vi "Fetch VI Method Info.vi"(7 "Fetch FP Info? (F)":bool, 8 "Error in":errorcluster caption="Error in (no error)", 9 "Dispatch (None)":T4, 10 "VI Reference":refnum<vi>, 11 "VI ProjectItem in":refnum<vi>) -> (0 "Error out":errorcluster, 3 "Method Spec Cluster":T1)   [LabVIEW 2023, in "VIDoc Parsing.lvlib"]
uses:
  VIDoc Parsing.lvlib
  TypeDefs/Class Dispatch Type Enum.ctl
  TypeDefs/Method Spec Cluster.ctl
  TypeDefs/VI Type Extended Enum.ctl
  <vilib>/picture/picture.llb/imagedata.ctl
  TypeDefs/Controls Info Cluster.ctl
  <vilib>/Utility/miscctls.llb/LVKeyTypeDef.ctl
  <vilib>/Utility/miscctls.llb/LVPointTypeDef.ctl
  Structure Reporter/Tree Cluster.ctl
  Structure Reporter/Structure Reporter.lvlib
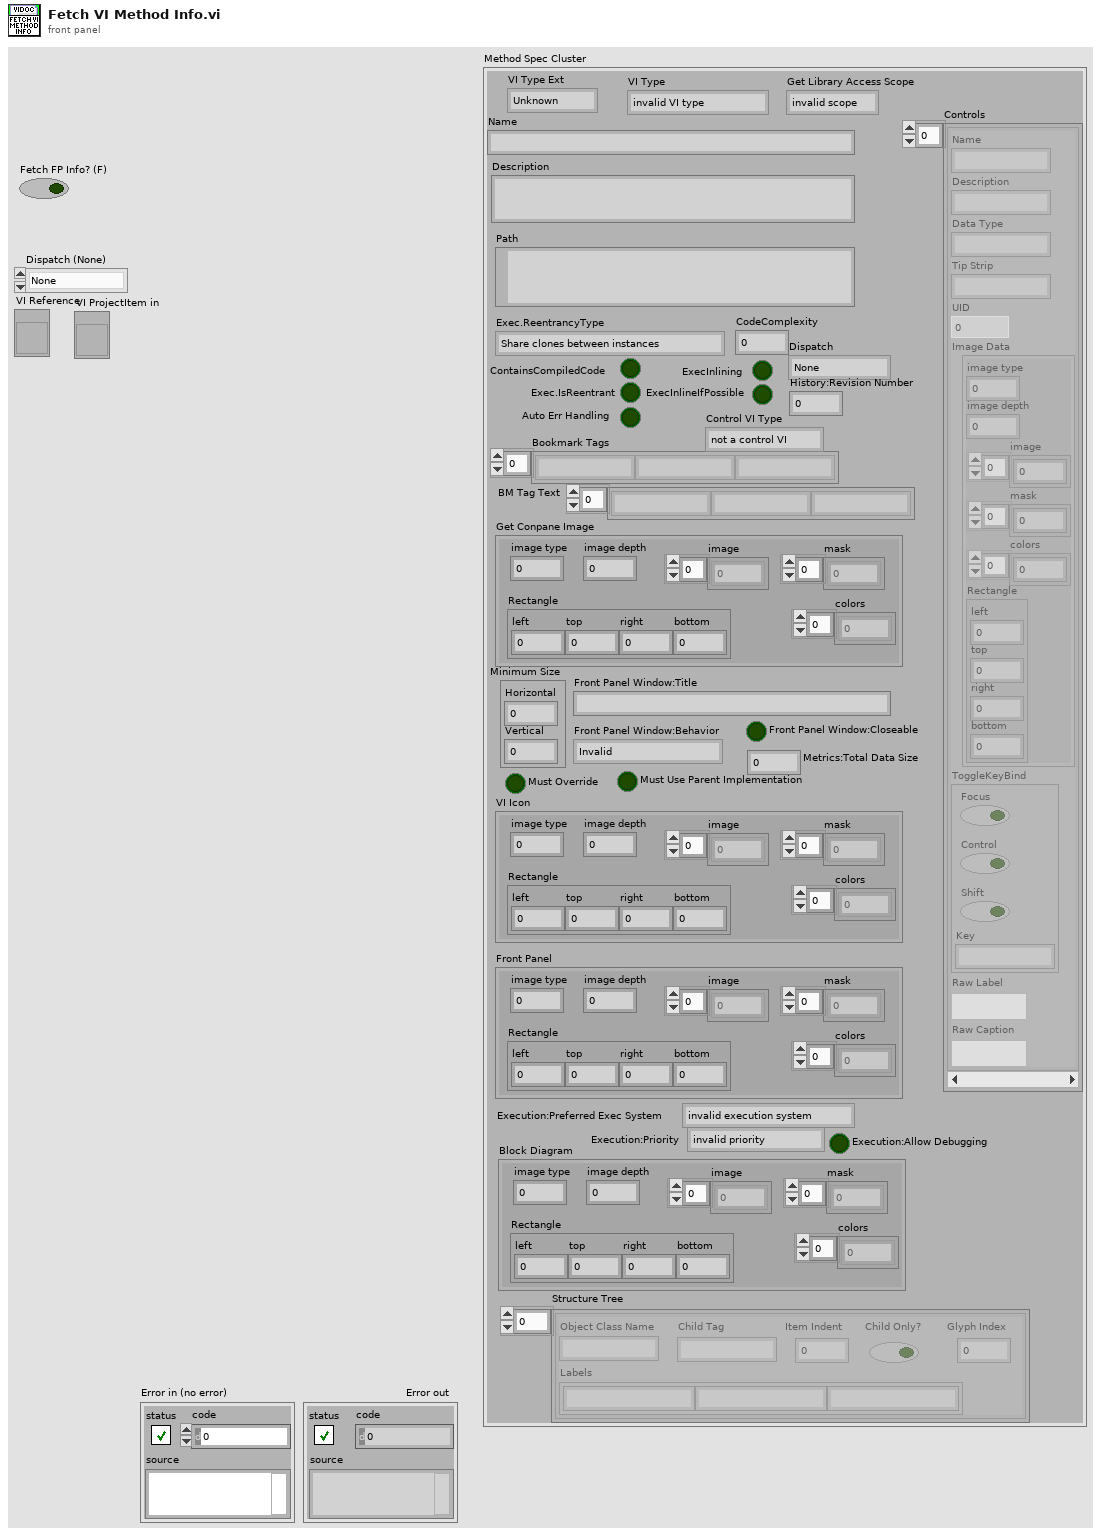
[diagram p1: front panel]
types:
  T1 = typedef "VIDoc Parsing.lvlib/Method Spec Cluster.ctl" = cluster{"VI Type Ext":T2, "Name":string, "Path":path, "Get Conpane Image":T3, "Description":string, "Get Library Access Scope":enum32{"invalid scope", "public", "private", "protected", "community"}, "Dispatch":T4, "ContainsCompiledCode":bool, "Exec.IsReentrant":bool, "Exec.ReentrancyType":enum16{"Share clones between instances", "Preallocate clone for each instance"}, "ExecInlining":bool, "ExecInlineIfPossible":bool, "Auto Err Handling":bool, "CodeComplexity":sgl, "Bookmark Tags":string[], "Control VI Type":enum32{"not a control VI", "control", "typedef", "strict typedef"}, "Controls":T5[], "VI Type":enum32{"invalid VI type", "Standard VI", "Control VI", "Global VI", "Polymorphic VI", "Configuration VI", "SubSystem", "Facade VI", "Method VI", "Statechart Diagram VI"}, "Minimum Size":T7, "Front Panel Window:Title":string, "Front Panel Window:Behavior":enum32{"Invalid", "Default", "Floating", "Floating/Auto-Hide", "Modal"}, "Front Panel Window:Closeable":bool, "Must Override":bool, "Must Use Parent Implementation":bool, "VI Icon":T3, "Front Panel":T3, "History:Revision Number":u32, "Metrics:Total Data Size":u32, "Execution:Allow Debugging":bool, "Execution:Preferred Exec System":enum32{"invalid execution system", "user interface", "standard", "instrument i/o", "data acquisition", "other 1", "other 2", "same as caller"}, "Execution:Priority":enum32{"invalid priority", "background priority", "normal priority", "above normal priority", "high priority", "time critical priority", "subroutine"}, "BM Tag Text":string[], "Block Diagram":T3, "Structure Tree":T8[]}
  T2 = typedef "VIDoc Parsing.lvlib/VI Type Extended Enum.ctl" = enum16{"Unknown", "Class Method", "Class Accessor Get", "Class Accessor Set", "Class Control", "Library Method", "Library Control", "VI", "Control"}
  T3 = typedef "imagedata.ctl" = cluster{"image type":i32, "image depth":i32, "image":u8[], "mask":u8[], "colors":u32[], "Rectangle":cluster{"left":i16, "top":i16, "right":i16, "bottom":i16}}
  T4 = typedef "VIDoc Parsing.lvlib/Class Dispatch Type Enum.ctl" = enum16{"None", "Static", "Dynamic"}
  T5 = typedef "VIDoc Parsing.lvlib/Controls Info Cluster.ctl" = cluster{"Name":string, "Description":string, "Data Type":string, "Tip Strip":string, "UID":i32, "Image Data":T3, "ToggleKeyBind":T6, "Raw Label":string, "Raw Caption":string}
  T6 = typedef "LVKeyTypeDef.ctl" = cluster{"Focus":bool, "Control":bool, "Shift":bool, "Key":string}
  T7 = typedef "LVPointTypeDef.ctl" = cluster{"Horizontal":i16, "Vertical":i16}
  T8 = typedef "VIDoc Parsing.lvlib/Structure Reporter.lvlib/Tree Cluster.ctl" = cluster{"Object Class Name":string, "Labels":string[], "Child Tag":string, "Item Indent":i32, "Child Only?":bool, "Glyph Index":i32}
  T9 = enum32{"not a control VI", "control", "typedef", "strict typedef"}
  T10 = enum16{"Share clones between instances", "Preallocate clone for each instance"}
  T11 = enum32{"invalid execution system", "user interface", "standard", "instrument i/o", "data acquisition", "other 1", "other 2", "same as caller"}
  T12 = enum32{"invalid priority", "background priority", "normal priority", "above normal priority", "high priority", "time critical priority", "subroutine"}
  T13 = enum32{"invalid scope", "public", "private", "protected", "community"}
  T14 = typedef "LVBookmarkInfoTypeDef.ctl" = cluster{"Bookmark ID":u32, "Bookmark Tag":string, "Label Text":string}[]
  T15 = typedef "VIDoc Parsing.lvlib/Structure Reporter.lvlib/Structure Result 2.ctl" = cluster{"Depth":i32, "Top":i32, "Left":i32, "Frame index":i32, "Struct":i32, "Object Class Name":string, "Object UID":i32, "Label Visible":bool, "Object Label":string, "SD Label Visible":bool, "Object SD Label":string, "Frame Name":string, "Diag UID":i32, "Owner Class Name":string, "Owner UID":i32, "Diag Struct":i32[], "Parent Struct":i32, "Diag UIDs":i32[], "Tree Name":string, "Diag Ref":refnum<vi>, "Owner Classes":string[], "Owner":refnum<vi>, "Owner UIDs":i32[], "Tag Indent":i32, "Tag Value":i32, "Child Tag":string}
  T16 = enum32{"Invalid", "Default", "Floating", "Floating/Auto-Hide", "Modal"}
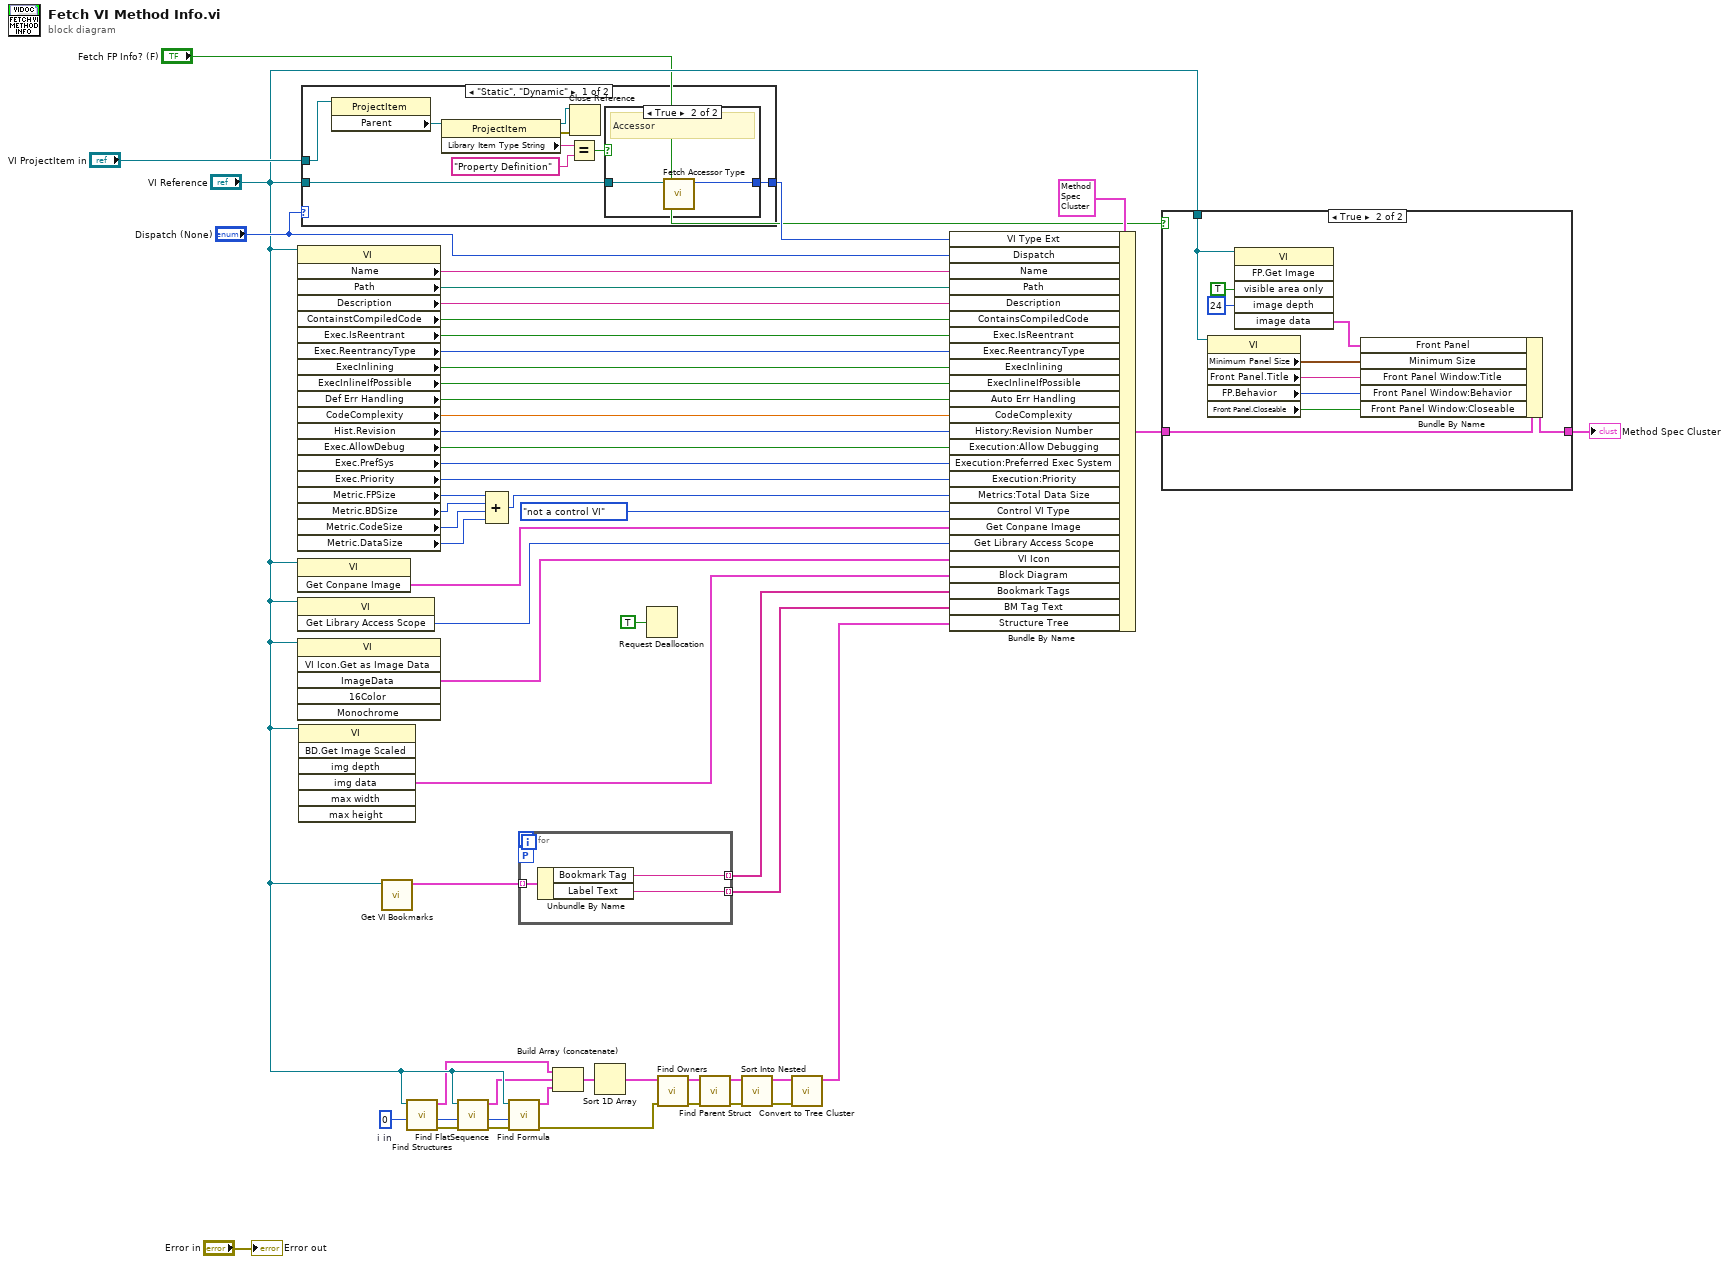
[diagram p0: block diagram]
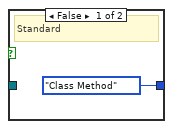
[diagram p3: hidden frame]
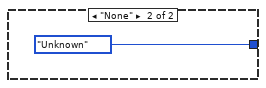
[diagram p4: hidden frame]
diagram:
  w17 = 0  # i in
  n1 = property class="VI"(reference="VI Reference") -> ("Name"=w48:string, "Path"=w47:path, "Description"=w46:string, "ContainstCompiledCode"=w45:bool, "Exec.IsReentrant"=w44:bool, "Exec.ReentrancyType"=w43:T10, "ExecInlining"=w42:bool, "ExecInlineIfPossible"=w41:bool, "Def Err Handling"=w40:bool, "CodeComplexity"=w39:sgl, "Hist.Revision"=w38:u32, "Exec.AllowDebug"=w37:bool, "Exec.PrefSys"=w36:T11, "Exec.Priority"=w35:T12, "Metric.FPSize"=w53:u32, "Metric.BDSize"=w52:u32, "Metric.CodeSize"=w51:u32, "Metric.DataSize"=w50:u32)  [unwired: 1 in, 2 out]
  n2 = invoke class="VI" method="Get Conpane Image"(reference="VI Reference") -> ("Get Conpane Image"=w33:T3)  [unwired: 2 in, 2 out]
  n3 = invoke class="VI" method="Get Library Access Scope"(reference="VI Reference") -> ("Get Library Access Scope"=w32:T13)  [unwired: 2 in, 2 out]
  n4 = invoke class="VI" method="VI Icon.Get as Image Data"(reference="VI Reference") -> ("ImageData"=w31:T3)  [unwired: 5 in, 5 out]
  n5 = invoke class="VI" method="BD.Get Image Scaled"(reference="VI Reference") -> ("img data"=w21:T3)  [unwired: 6 in, 6 out]
  n6 = case shown="\"Static\", \"Dynamic\"" "Dispatch (None)" {
    tunnel: "VI ProjectItem in" -> [w64 _]
    tunnel: [w60 VI_Type_Extended_Enum."Unknown" ("VI Type Ext")] -> w28
    tunnel: "VI Reference" -> [w58 _]
    frame "Static", "Dynamic" {
      n7 = property class="ProjectItem"(reference=w64) -> ("Parent"=w61:refnum<vi>)  [unwired: 1 in, 2 out]
      n8 = property class="ProjectItem"(reference=w61) -> (reference out=w56:refnum<vi>, error out=w57:errorcluster, "Library Item Type String"=w62:string)  [unwired: 1 in]
      n9 = Equal?(x=w62, y="Property Definition") -> (x = y?=w59:bool)
      n10 = Close Reference(reference=w56, error in (no error)=w57) -> ()  [unwired: 1 out]
      n11 = case shown="True" w59 {
        tunnel: [VI_Type_Extended_Enum."Class Method" w66] -> w60
        tunnel: w58 -> [_ w67]
        frame False {
          # "Standard"
        }
        frame True {
          # "Accessor"
          n12 = call "Fetch Accessor Type.vi"("VI in"=w67) -> ("VI Type Ext"=w66:T2)  [unwired: 9 in, 1 out]
        }
      }
    }
    frame "None" {
    }
  }
  n13 = call "Get VI Bookmarks.vi"("VI in"="VI Reference") -> ("BookmarkInfo"=w27:T14)  [unwired: 9 in, 1 out]
  n14 = call "Find Structures.vi"("i in"=w17, "VI in"="VI Reference") -> ("error out"=w4:errorcluster, "i out"=w16:i32, "Structures"=w18:T15[])  [unwired: 7 in]
  n15 = call "Find FlatSequence.vi"("error in (no error)"=w4, "i in"=w16, "VI in"="VI Reference") -> ("error out"=w3:errorcluster, "i out"=w13:i32, "FlatSequences"=w15:T15[])  [unwired: 6 in]
  n16 = Compound Arithmetic op=ADD(w53, w52, w51, w50) -> (w34:u32)
  n17 = call "Find Formula.vi"("error in (no error)"=w3, "i in"=w13, "VI in"="VI Reference") -> ("error out"=w2:errorcluster, "Array"=w14:T15[])  [unwired: 6 in, 1 out]
  n18 = for {
    tunnel: w27 -> [w71] mode=indexing
    tunnel: [w70] -> w26 mode=indexing
    workers-P: _ -> [_]
    tunnel: [w69] -> w25 mode=indexing
    n19 = Unbundle By Name(w71) -> ("Bookmark Tag"=w70:string, "Label Text"=w69:string)
  }
  n20 = Build Array (concatenate)(w18, w15, w14) -> (w12:T15[])
  n21 = Sort 1D Array(array=w12) -> (sorted array=w11:T15[])
  n22 = Request Deallocation(TRUE ("flag")) -> ()
  n23 = call "Find Owners.vi"("error in (no error)"=w2, "Array in"=w11) -> ("error out"=w9:errorcluster, "Array out"=w10:T15[])  [unwired: 8 in]
  n24 = call "Find Parent Struct.vi"("error in (no error)"=w9, "Objects in"=w10) -> ("error out"=w7:errorcluster, "Found Parent Struct"=w8:T15[])  [unwired: 8 in]
  n25 = call "Sort Into Nested.vi"("error in (no error)"=w7, "Found Parent Struct"=w8) -> ("error out"=w6:errorcluster, "Nested Structures"=w5:T15[])  [unwired: 8 in]
  n26 = call "Convert to Tree Cluster.vi"("error in (no error)"=w6, "Array in"=w5) -> ("Array out"=w20:T8[])  [unwired: 8 in, 1 out]
  n27 = Bundle By Name(cluster=T1 {"VI Type Ext"=enum."Unknown", "Name"="", "Path"=path "", "Get Conpane Image"={"image type"=0, "image depth"=0, "image"=[], "mask"=[], "colors"=[], "Rectangle"={"left"=0, "top"=0, "right"=0, "bottom"=0}}, "Description"="", "Get Library Access Scope"=enum."invalid scope", "Dispatch"=enum."None", "ContainsCompiledCode"=FALSE, "Exec.IsReentrant"=FALSE, "Exec.ReentrancyType"=enum."Share clones between instances", "ExecInlining"=FALSE, "ExecInlineIfPossible"=FALSE, "Auto Err Handling"=FALSE, "CodeComplexity"=0.0, "Bookmark Tags"=[], "Control VI Type"=enum."not a control VI", "Controls"=[], "VI Type"=enum."invalid VI type", "Minimum Size"={"Horizontal"=0, "Vertical"=0}, "Front Panel Window:Title"="", "Front Panel Window:Behavior"=enum."Invalid", "Front Panel Window:Closeable"=FALSE, "Must Override"=FALSE, "Must Use Parent Implementation"=FALSE, "VI Icon"={"image type"=0, "image depth"=0, "image"=[], "mask"=[], "colors"=[], "Rectangle"={"left"=0, "top"=0, "right"=0, "bottom"=0}}, "Front Panel"={"image type"=0, "image depth"=0, "image"=[], "mask"=[], "colors"=[], "Rectangle"={"left"=0, "top"=0, "right"=0, "bottom"=0}}, "History:Revision Number"=0, "Metrics:Total Data Size"=0, "Execution:Allow Debugging"=FALSE, "Execution:Preferred Exec System"=enum."invalid execution system", "Execution:Priority"=enum."invalid priority", "BM Tag Text"=[], "Block Diagram"={"image type"=0, "image depth"=0, "image"=[], "mask"=[], "colors"=[], "Rectangle"={"left"=0, "top"=0, "right"=0, "bottom"=0}}, "Structure Tree"=[]}, "VI Type Ext"=w28, "Dispatch"="Dispatch (None)", "Name"=w48, "Path"=w47, "Description"=w46, "ContainsCompiledCode"=w45, "Exec.IsReentrant"=w44, "Exec.ReentrancyType"=w43, "ExecInlining"=w42, "ExecInlineIfPossible"=w41, "Auto Err Handling"=w40, "CodeComplexity"=w39, "History:Revision Number"=w38, "Execution:Allow Debugging"=w37, "Execution:Preferred Exec System"=w36, "Execution:Priority"=w35, "Metrics:Total Data Size"=w34, "Control VI Type"=T9."not a control VI", "Get Conpane Image"=w33, "Get Library Access Scope"=w32, "VI Icon"=w31, "Block Diagram"=w21, "Bookmark Tags"=w26, "BM Tag Text"=w25, "Structure Tree"=w20) -> (w24:T1)
  n28 = case shown="True" "Fetch FP Info? (F)" {
    tunnel: [w72 w82] -> w55
    tunnel: w24 -> [w72 w81]
    tunnel: "VI Reference" -> [_ w80]
    frame False {
    }
    frame True {
      n29 = property class="VI"(reference=w80) -> ("Minimum Panel Size"=w79:T7, "Front Panel.Title"=w75:string, "FP.Behavior"=w74:T16, "Front Panel.Closeable"=w73:bool)  [unwired: 1 in, 2 out]
      n30 = invoke class="VI" method="FP.Get Image"(reference=w80, "visible area only"=TRUE ("Visible Area Only"), "image depth"=24 ("Image Depth")) -> ("image data"=w76:T3)  [unwired: 3 in, 5 out]
      n31 = Bundle By Name(cluster=w81, "Front Panel"=w76, "Minimum Size"=w79, "Front Panel Window:Title"=w75, "Front Panel Window:Behavior"=w74, "Front Panel Window:Closeable"=w73) -> (w82:T1)
    }
  }
  "Method Spec Cluster" <- w55
  "Error out" <- "Error in"
